vi "test-runnee.vi"() -> (0 "errors":errorcluster[](array[cluster]))   [LabVIEW 2020]
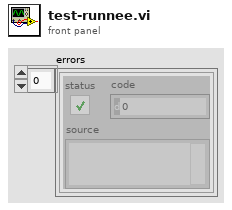
[diagram p1: front panel]
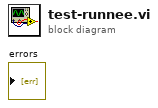
[diagram p0: block diagram]
diagram:
